vi "Move Weave to Limit Switch.vi"(10 "Call Mode":enum16{"Synchronous", "Asynchronous"}(ring), 11 "Switch":enum16{"Lower Switch", "Upper Switch"}(ring)) -> ()   [LabVIEW 2015]
uses:
  Robot Global Data.vi
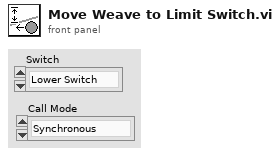
[diagram p1: front panel]
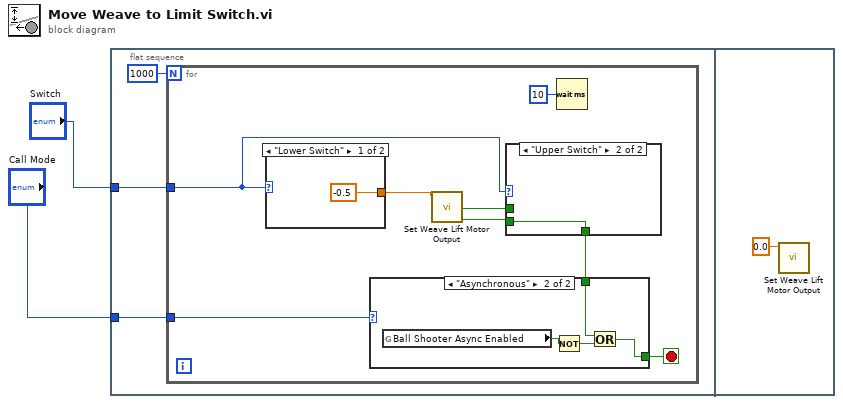
[diagram p0: block diagram]
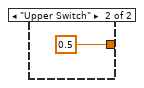
[diagram p4: hidden frame]
diagram:
  n1 = flat-sequence {
    tunnel: "Switch" -> [w4]
    tunnel: "Call Mode" -> [w3]
    frame #0 {
      n2 = for {
        N: 1000 -> [_]
        tunnel: w4 -> [w12]
        tunnel: w3 -> [w11]
        stop <- w10 stop-if-true
        n3 = case shown="\"Lower Switch\"" w12 {
          tunnel: [-0.5 0.5] -> w8
          frame "Lower Switch" {
          }
          frame "Upper Switch" {
          }
        }
        n4 = call "Set Weave Lift Motor Output.vi"("Output"=w8) -> ("Upper Switch Pressed"=w6:bool, "Lower Switch Pressed"=w7:bool)  [unwired: 1 out]
        n5 = case shown="\"Upper Switch\"" w12 {
          tunnel: [w19 w20] -> w9
          tunnel: w7 -> [w19 _]
          tunnel: w6 -> [_ w20]
          frame "Lower Switch" {
          }
          frame "Upper Switch" {
          }
        }
        n6 = case shown="\"Asynchronous\"" w11 {
          tunnel: [w14 w16] -> w10
          tunnel: w9 -> [w14 w18]
          frame "Synchronous" {
          }
          frame "Asynchronous" {
            n7 = global read "Robot Global Data.vi" "Ball Shooter Async Enabled"() -> (w17:bool)
            n8 = Not(x=w17) -> (.not. x?=w15:bool)
            n9 = Or(x=w18, y=w15) -> (x .or. y?=w16:bool)
          }
        }
        n10 = Wait (ms)(milliseconds to wait=u32 10) -> ()  [unwired: 1 out]
      }
    }
    frame #1 {
      n11 = call "Set Weave Lift Motor Output.vi"("Output"=0.0) -> ()  [unwired: 3 out]
    }
  }
